vi "MoAgSy_Host_GPG_cryption.vi"(0 "Host_Reference":refnum<class "HGF_Reference.lvclass">, 3 "string in":string, 5 "error in (no error)":errorcluster, 6 "timeout in ms (-1)":i32=-1, 7 "reveicer array":string[](array[string]), 8 "task":enum16{"encrypt", "decrypt", "sign", "verify"}(ring), 9 "receiver":string) -> (13 "success":bool, 14 "dup Host_Reference":refnum<class "HGF_Reference.lvclass">, 17 "String out":string, 19 "error out":errorcluster)   [LabVIEW 2009, in "MoAgSy.lvlib" / "MoAgSy_Host.lvclass"]
uses:
  MoAgSy_Host.lvclass
  HGF_BaseClasses/HGF_Reference/HGF_Reference.lvclass
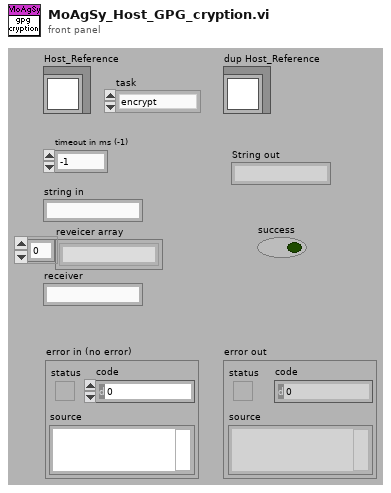
[diagram p1: front panel]
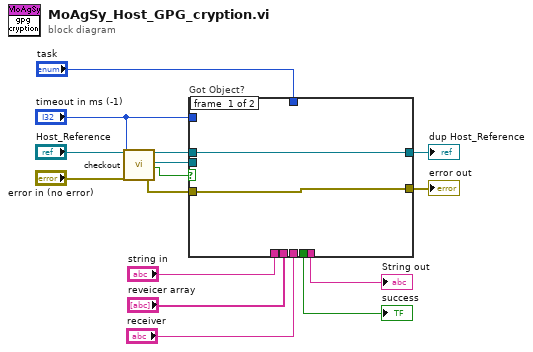
[diagram p0: block diagram]
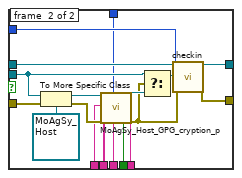
[diagram p2: hidden frame]
diagram:
  n1 = call "checkout.vi"("HGF_Reference"="Host_Reference", "timeout in ms (-1)"="timeout in ms (-1)", "error in (no error)"="error in (no error)") -> ("dup HGF_Reference"=w10:refnum<class "HGF_Reference.lvclass">, "Object"=w13:refnum<class>, "got object?"=w11:bool, "error out"=w14:errorcluster)  [unwired: 13 out]
  n2 = case "Got Object?" shown="True" w11 {
    tunnel: w14 -> [w16 w35]
    tunnel: w13 -> [_ w29]
    tunnel: w10 -> [w17 w33]
    tunnel: [w17 w32] -> w9
    tunnel: "timeout in ms (-1)" -> [_ w31]
    tunnel: [w16 w30] -> w7
    tunnel: [_ w23] -> w6
    tunnel: [_ w22] -> w5
    tunnel: "receiver" -> [_ w21]
    tunnel: "reveicer array" -> [_ w20]
    tunnel: "task" -> [_ w19]
    tunnel: "string in" -> [_ w18]
    frame #0 {
    }
    frame #1 {
      n3 = To More Specific Class(target class=refnum<class "MoAgSy_Host.lvclass"> refnum ("MoAgSy.lvlib:MoAgSy_Host.lvclass"), reference=w29, error in=w35) -> (specific class reference=w27:refnum<class "MoAgSy_Host.lvclass">, error out=w25:errorcluster)
      n4 = call "MoAgSy_Host_GPG_cryption_p.vi"("MoAgSy_Host"=w27, "string in"=w18, "error IO"=w25, "reveicer array"=w20, "task"=w19, "receiver"=w21) -> ("success"=w22:bool, "dup MoAgSy_Host"=w26:refnum<class "MoAgSy_Host.lvclass">, "String out"=w23:string, "error out"=w24:errorcluster)  [unwired: 10 in]
      n5 = Select(t=w29, s=w24, f=w26) -> (s? t:f=w28:refnum<class>)
      n6 = call "checkin.vi"("HGF_Reference"=w33, "Object"=w28, "timeout /ms (-1)"=w31, "error in (no error)"=w24) -> ("dup HGF_Reference"=w32:refnum<class "HGF_Reference.lvclass">, "error out"=w30:errorcluster)  [unwired: 14 out]
    }
  }
  "dup Host_Reference" <- w9
  "error out" <- w7
  "String out" <- w6
  "success" <- w5
